vi "Build Monitor Waveform.vi"(8 "error in (no error)":errorcluster, 11 "Queue Elements":T1[](array[typedef])) -> (0 "error out":errorcluster, 3 "Digital Data Table":digitaldata)   [LabVIEW 2016]
uses:
  Typedefs/Monitor Data Element.ctl
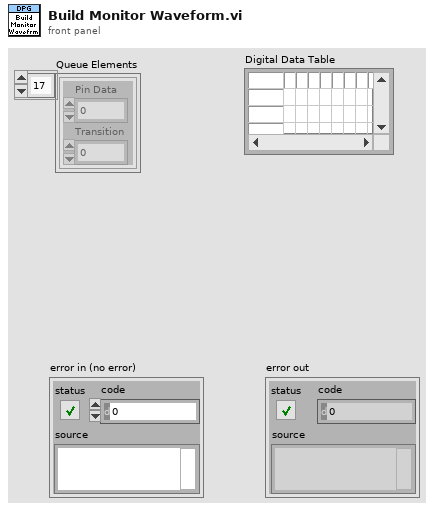
[diagram p1: front panel]
types:
  T1 = typedef "Monitor Data Element.ctl" = cluster{"Pin Data":u32, "Transition ":u32}
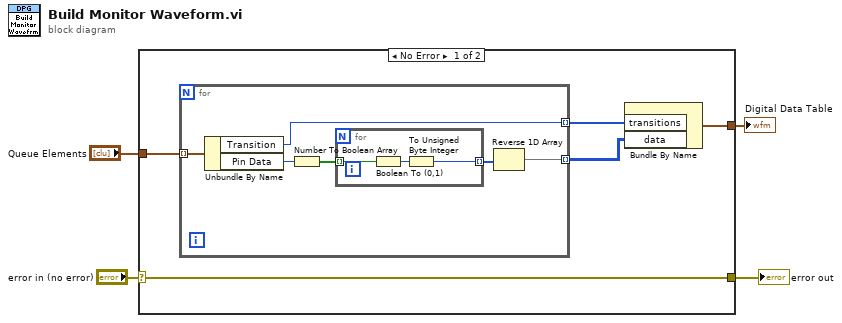
[diagram p0: block diagram]
diagram:
  n1 = case shown="No Error" "error in (no error)" {
    selector: "error in (no error)" -> [w5 w19]
    tunnel: "Queue Elements" -> [w9 _]
    tunnel: [w6 _] -> w2
    tunnel: [w5 w19] -> w1
    frame No Error {
      n2 = for {
        tunnel: w9 -> [w15] mode=indexing
        tunnel: [w12] -> w8 mode=indexing
        tunnel: [w10] -> w7 mode=indexing
        n3 = Unbundle By Name(w15) -> ("Transition"=w12:u32, "Pin Data"=w14:u32)
        n4 = Number To Boolean Array(number=w14) -> (Boolean array=w13:bool[])
        n5 = for {
          tunnel: w13 -> [w18] mode=indexing
          tunnel: [w16] -> w11 mode=indexing
          n6 = Boolean To (0,1)(Boolean=w18) -> (0, 1=w17:i16)
          n7 = To Unsigned Byte Integer(number=w17) -> (unsigned 8bit integer=w16:u8)
        }
        n8 = Reverse 1D Array(array=w11) -> (reversed array=w10:u8[])
      }
      n9 = Bundle By Name("transitions"=w8, "data"=w7) -> (w6:digitaldata)  [unwired: 1 in]
    }
    frame Error {
    }
  }
  "error out" <- w1
  "Digital Data Table" <- w2
